vi "ConvertSenseChannelToSenseNumber.vi"(11 "Channel (1 or 2)":u8 min=1 max=2 step=1) -> (3 "Sense Number":string)   [LabVIEW 2009, in "Keithley-6482-Visa.lvlib"]
uses:
  <instrlib>/Keithley-6482-Visa9.0/Keithley-6482-Visa.lvlib
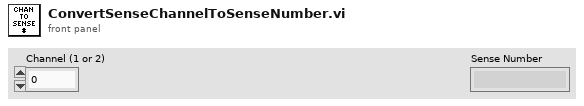
[diagram p1: front panel]
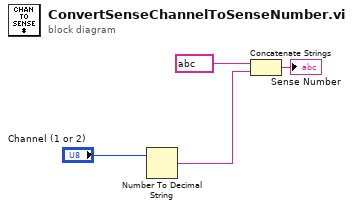
[diagram p0: block diagram]
diagram:
  n1 = Number To Decimal String(number="Channel (1 or 2)") -> (decimal integer string=w2:string)  [unwired: 1 in]
  n2 = Concatenate Strings(string ?, w2) -> (→"Sense Number":string)
